vi "Send Output Vals Using Tags.vi"(0 "Message Handler Loop Data in":T2, 5 "[Parsed Tags]":T1[](array[typedef]), 7 "Array of VData in":variant[](array[variant]), 11 "error in (no error)":errorcluster) -> (15 "error out":errorcluster)   [LabVIEW 2018]
doc: "Writes output values bases on the input tag information and variant values. The variant values must be in the right format to match the named tag, or an error will occur.\n\nWarning: A boolean output sent with an analog output card, must be converted to a numeric value before being put through this VI because the analog output data will not understand a boolean input."
uses:
  RT - Instrument IO.lvlib
  Private Controls/Message Handler Loop Data.ctl
  Top Level/Shared Controls/Parsed Tag Cluster.ctl
  FPGA/FPGA VI Reference.ctl
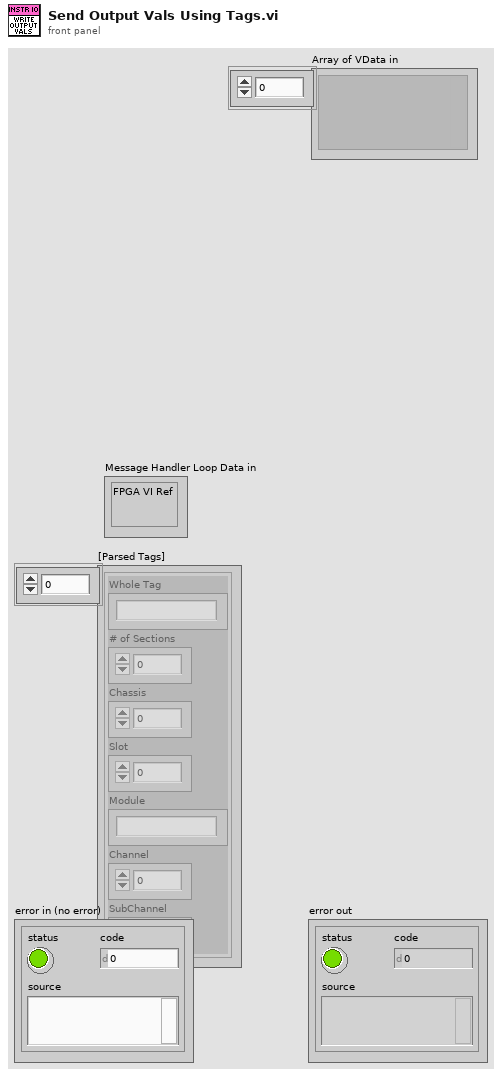
[diagram p1: front panel]
types:
  T1 = typedef "Parsed Tag Cluster.ctl" = cluster{"Whole Tag":string, "# of Sections":u8, "Chassis":u8, "Slot":u8, "Module":string, "Channel":u8, "SubChannel":u8}
  T2 = typedef "RT - Instrument IO.lvlib/Message Handler Loop Data.ctl" = cluster{"FPGA VI Ref":T3}
  T3 = typedef "FPGA VI Reference.ctl" = refnum<k20>
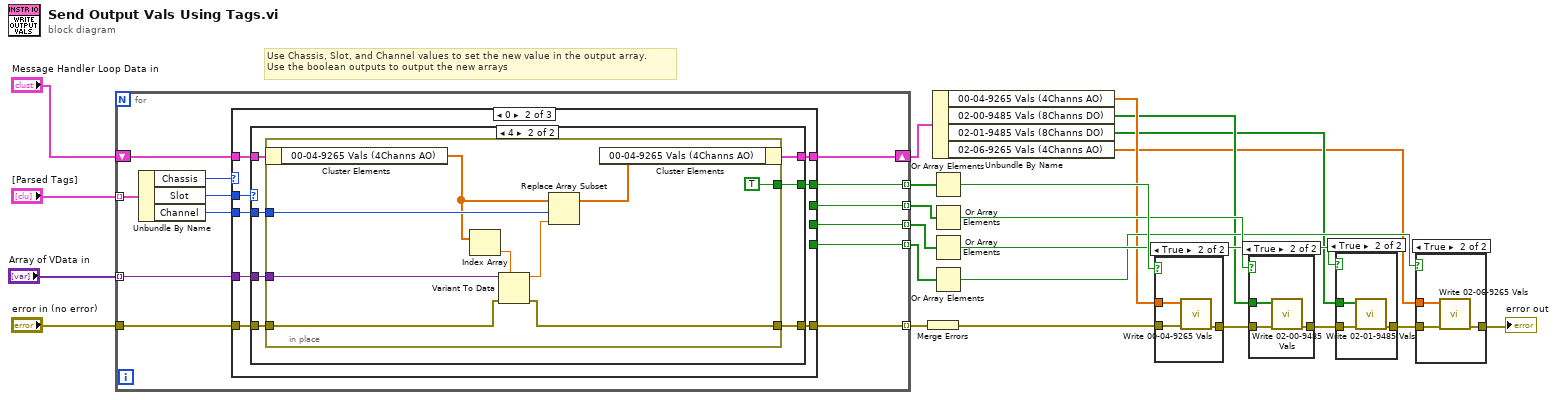
[diagram p0: block diagram]
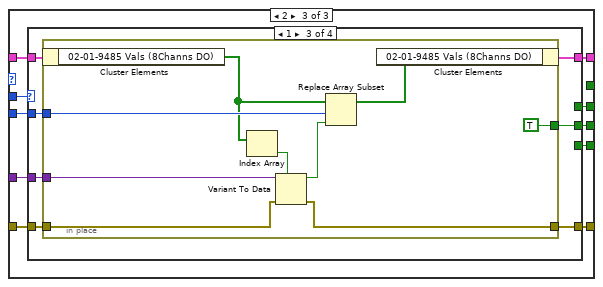
[diagram p8: hidden frame]
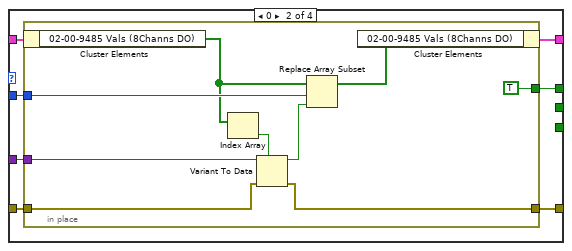
[diagram p10: hidden frame]
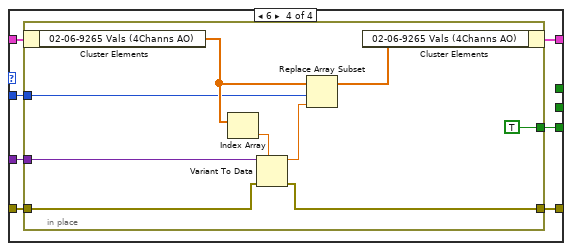
[diagram p11: hidden frame]
diagram:
  # "Use Chassis, Slot, and Channel values to set the new value in the output array.\nUse the boolean outputs to output the new arrays"
  n1 = for {
    tunnel: "error in (no error)" -> [w35]
    tunnel: "[Parsed Tags]" -> [w36] mode=indexing
    tunnel: [w32] -> w22 mode=indexing
    tunnel: "Array of VData in" -> [w29] mode=indexing
    shift-right: [w28] -> w14
    shift-left: "Message Handler Loop Data in" -> [w30]
    tunnel: [w27] -> w18 mode=indexing
    tunnel: [w26] -> w17 mode=indexing
    tunnel: [w25] -> w16 mode=indexing
    tunnel: [w24] -> w15 mode=indexing
    n2 = Unbundle By Name(w36) -> ("Chassis"=w34:u8, "Slot"=w33:u8, "Channel"=w31:u8)
    n3 = case shown="0" w34 {
      tunnel: w35 -> [w38 w45 w73]
      tunnel: w33 -> [_ w44 w72]
      tunnel: [w38 w46 w74] -> w32
      tunnel: w31 -> [_ w43 w71]
      tunnel: w30 -> [w37 w42 w70]
      tunnel: w29 -> [_ w41 w69]
      tunnel: [w37 w40 w68] -> w28
      tunnel: [_ w39 _] -> w27
      tunnel: [_ _ w67] -> w26
      tunnel: [_ _ w66] -> w25
      tunnel: [_ _ w65] -> w24
      frame Default {
      }
      frame 0 {
        n4 = case shown="4" w44 {
          tunnel: [w48 w52] -> w46
          tunnel: w45 -> [w48 w53]
          tunnel: w43 -> [_ w55]
          tunnel: w42 -> [w47 w51]
          tunnel: w41 -> [_ w54]
          tunnel: [w47 w50] -> w40
          tunnel: [_ w49] -> w39
          frame Default {
          }
          frame 4 {
            n5 = in-place {
              in-place-border: w55 -> [w64]
              in-place-border: w54 -> [w62]
              in-place-border: w53 -> [w61]
              in-place-border: [w60] -> w52
              in-place-border: [TRUE] -> w49
              n6 = in-place-cluster #1(w51) -> ("00-04-9265 Vals (4Channs AO)"=w58:sgl[])
              n7 = Index Array(array=w58) -> (element=w63:sgl)  [unwired: 1 in]
              n8 = Variant To Data(error in=w61, type=w63, Variant=w62) -> (data=w59:sgl, error out=w60:errorcluster)
              n9 = Replace Array Subset(array=w58, new element=w59, index=w64) -> (w57:sgl[])
              n10 = in-place-cluster #1("00-04-9265 Vals (4Channs AO)"=w57) -> (w50:T2)
            }
          }
        }
      }
      frame 2 {
        n11 = case shown="1" w72 {
          tunnel: [w76 w80 w96 w112] -> w74
          tunnel: w73 -> [w76 w81 w97 w113]
          tunnel: w71 -> [_ w83 w99 w115]
          tunnel: w70 -> [w75 w79 w95 w111]
          tunnel: w69 -> [_ w82 w98 w114]
          tunnel: [w75 w78 w94 w110] -> w68
          tunnel: [_ w77 _ _] -> w67
          tunnel: [_ _ w93 _] -> w66
          tunnel: [_ _ _ w109] -> w65
          frame Default {
          }
          frame 0 {
            n12 = in-place {
              in-place-border: w83 -> [w92]
              in-place-border: w82 -> [w90]
              in-place-border: w81 -> [w89]
              in-place-border: [w88] -> w80
              in-place-border: [TRUE] -> w77
              n13 = in-place-cluster #2(w79) -> ("02-00-9485 Vals (8Channs DO)"=w86:bool[])
              n14 = Index Array(array=w86) -> (element=w91:bool)  [unwired: 1 in]
              n15 = Variant To Data(error in=w89, type=w91, Variant=w90) -> (data=w87:bool, error out=w88:errorcluster)
              n16 = Replace Array Subset(array=w86, new element=w87, index=w92) -> (w85:bool[])
              n17 = in-place-cluster #2("02-00-9485 Vals (8Channs DO)"=w85) -> (w78:T2)
            }
          }
          frame 1 {
            n18 = in-place {
              in-place-border: w99 -> [w108]
              in-place-border: w98 -> [w106]
              in-place-border: w97 -> [w105]
              in-place-border: [w104] -> w96
              in-place-border: [TRUE] -> w93
              n19 = in-place-cluster #3(w95) -> ("02-01-9485 Vals (8Channs DO)"=w102:bool[])
              n20 = Index Array(array=w102) -> (element=w107:bool)  [unwired: 1 in]
              n21 = Variant To Data(error in=w105, type=w107, Variant=w106) -> (data=w103:bool, error out=w104:errorcluster)
              n22 = Replace Array Subset(array=w102, new element=w103, index=w108) -> (w101:bool[])
              n23 = in-place-cluster #3("02-01-9485 Vals (8Channs DO)"=w101) -> (w94:T2)
            }
          }
          frame 6 {
            n24 = in-place {
              in-place-border: w115 -> [w116]
              in-place-border: w114 -> [w123]
              in-place-border: w113 -> [w122]
              in-place-border: [w121] -> w112
              in-place-border: [TRUE] -> w109
              n25 = in-place-cluster #4(w111) -> ("02-06-9265 Vals (4Channs AO)"=w119:dbl[])
              n26 = Index Array(array=w119) -> (element=w124:dbl)  [unwired: 1 in]
              n27 = Variant To Data(error in=w122, type=w124, Variant=w123) -> (data=w120:dbl, error out=w121:errorcluster)
              n28 = Replace Array Subset(array=w119, new element=w120, index=w116) -> (w118:dbl[])
              n29 = in-place-cluster #4("02-06-9265 Vals (4Channs AO)"=w118) -> (w110:T2)
            }
          }
        }
      }
    }
  }
  n30 = Merge Errors(w22) -> (w10:errorcluster)
  n31 = Unbundle By Name(w14) -> ("00-04-9265 Vals (4Channs AO)"=w4:sgl[], "02-00-9485 Vals (8Channs DO)"=w3:bool[], "02-01-9485 Vals (8Channs DO)"=w2:bool[], "02-06-9265 Vals (4Channs AO)"=w1:dbl[])
  n32 = Or Array Elements(Boolean array=w18) -> (logical OR=w8:bool)
  n33 = Or Array Elements(Boolean array=w17) -> (logical OR=w7:bool)
  n34 = Or Array Elements(Boolean array=w16) -> (logical OR=w6:bool)
  n35 = Or Array Elements(Boolean array=w15) -> (logical OR=w5:bool)
  n36 = case shown="True" w8 {
    tunnel: [w125 w128] -> w13
    tunnel: w10 -> [w125 w127]
    tunnel: w4 -> [_ w126]
    frame False {
    }
    frame True {
      n37 = call "Write 00-04-9265 Vals.vi"("error in (no error)"=w127, "Data (4Channs AO) (Empty: Default)"=w126) -> ("error out"=w128:errorcluster)  [unwired: 9 in]
    }
  }
  n38 = case shown="True" w7 {
    tunnel: w13 -> [w129 w132]
    tunnel: [w129 w131] -> w12
    tunnel: w3 -> [_ w130]
    frame False {
    }
    frame True {
      n39 = call "Write 02-00-9485 Vals.vi"("error in (no error)"=w132, "Data (8Channs DO) (Empty: Default)"=w130) -> ("error out"=w131:errorcluster)  [unwired: 9 in]
    }
  }
  n40 = case shown="True" w6 {
    tunnel: w12 -> [w133 w136]
    tunnel: [w133 w135] -> w11
    tunnel: w2 -> [_ w134]
    frame False {
    }
    frame True {
      n41 = call "Write 02-01-9485 Vals.vi"("error in (no error)"=w136, "Data (8Channs DO) (Empty: Default)"=w134) -> ("error out"=w135:errorcluster)  [unwired: 9 in]
    }
  }
  n42 = case shown="True" w5 {
    tunnel: w11 -> [w137 w140]
    tunnel: [w137 w139] -> w9
    tunnel: w1 -> [_ w138]
    frame False {
    }
    frame True {
      n43 = call "Write 02-06-9265 Vals.vi"("error in (no error)"=w140, "Data (4Channs AO) (Empty: Default)"=w138) -> ("error out"=w139:errorcluster)  [unwired: 9 in]
    }
  }
  "error out" <- w9
